vi "APU + 1 Directional Sim.vi"() -> ()   [LabVIEW 2013]
uses:
  IP Source/Version Token.ctl
  IP Source/APU/Settings.ctl
  IP Source/APU/Input.ctl
  IP Source/APU/Output.ctl
  IP Source/Directional Speed/Load Input.ctl
  IP Source/Directional Speed/Input.ctl
  IP Source/Directional Speed/Settings.ctl
  IP Source/APU/Shared Settings.ctl
  <vilib>/Platform/TimedLoop/XDataNode/timing_clust.ctl
  <vilib>/Platform/TimedLoop/XDataNode/nitl_modes.ctl
  <vilib>/Platform/TimedLoop/XDataNode/wakeup.ctl
  <vilib>/rvi/DataTransferAndStorage/Container/Common/niFpgaContainerGetUniqueNameForEmu.vi
  <vilib>/rvi/DataTransferAndStorage/Container/Common/niFpgaContainerSetEmuInfo.vi
  <vilib>/rvi/eio/common/nirviEmuReportErrorAndStop.vi
  <vilib>/rvi/Emulation/niFpgaSctlEmulationGetInTimedLoop.vi
  <vilib>/rvi/Emulation/niFpgaEmulationReportErrorSimple.vi
  <vilib>/rvi/Emulation/niFpgaGetClockAttributes.vi
  <vilib>/rvi/Emulation/niFpgaCriticalErrorInLSC.vi
  <vilib>/rvi/eio/common/nirviEmuTemplateMethod_errors.vi
  <vilib>/Platform/TimedLoop/XDataNode/XDataNode.xnode
  <vilib>/rvi/LocalResourceManager/LocalResourceManager.xnode
  <vilib>/eio/EIONode/EIONode.xnode
  <vilib>/Platform/TimedLoop/XDataNode/XDNodeRunTimeDep.lvlib
  IP Source/APU/APU.lvlib
  IP Source/Directional Speed/Directional Speed.lvlib
  IP Source/Engine Simulation Toolkit.lvlib
panel:
  in  "shared settings.my apu":T1 {"start" format="%#.15g"}
  in  "go.my apu":bool
  in  "settings.DirectionSim":T2
  in  "input.DirectionSim":T3
  in  "load input.DirectionSim":T4
  out "output.my apu":T5 caption="output"
  in  "input.my apu":T6={"desired speed"=0.0, "reset"=TRUE} caption="input"
  in  "settings.my apu":T7 caption="settings"
  in  "eps.version":T8
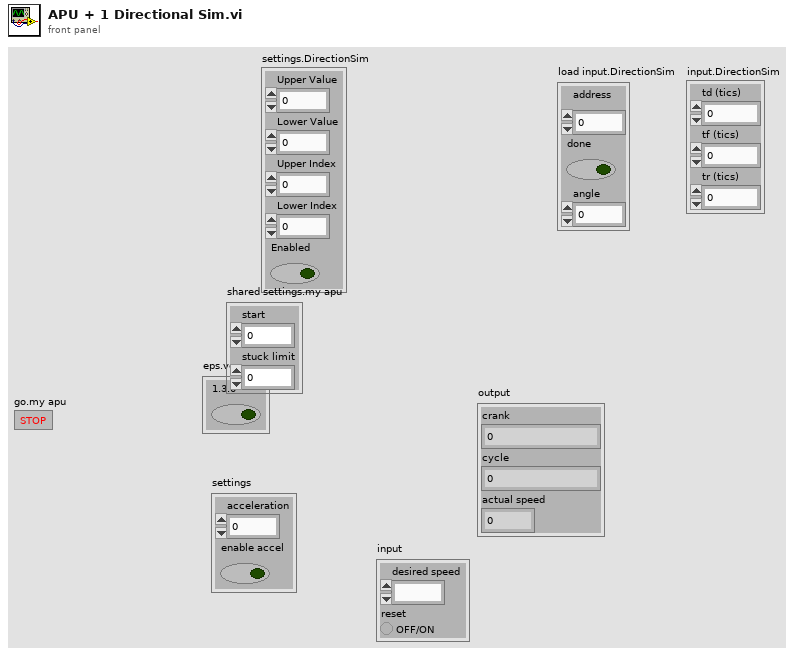
[diagram p1: front panel]
types:
  T1 = typedef "Engine Simulation Toolkit.lvlib/APU.lvlib/Shared Settings.ctl" = cluster{"start":fxp<+,17,17>, "stuck limit":fxp<+,18,18>}
  T2 = typedef "Engine Simulation Toolkit.lvlib/Directional Speed.lvlib/Settings.ctl" = cluster{"Upper Value":u16, "Lower Value":u16, "Upper Index":fxp<+,10,10>, "Lower Index":fxp<+,10,10>, "Enabled":bool}
  T3 = typedef "Engine Simulation Toolkit.lvlib/Directional Speed.lvlib/Input.ctl" = cluster{"td (tics)":u16, "tf (tics)":u16, "tr (tics)":u16}
  T4 = typedef "Engine Simulation Toolkit.lvlib/Directional Speed.lvlib/Load Input.ctl" = cluster{"address":fxp<+,10,10>, "done":bool, "angle":u16}
  T5 = typedef "Engine Simulation Toolkit.lvlib/APU.lvlib/Output.ctl" = cluster{"crank":u16, "cycle":u16, "actual speed":fxp<+/-,23,2>}
  T6 = typedef "Engine Simulation Toolkit.lvlib/APU.lvlib/Input.ctl" = cluster{"desired speed":fxp<+/-,23,2>, "reset":bool}
  T7 = typedef "Engine Simulation Toolkit.lvlib/APU.lvlib/Settings.ctl" = cluster{"acceleration":fxp<+,18,-20>, "enable accel":bool}
  T8 = typedef "Engine Simulation Toolkit.lvlib/Version Token.ctl" = cluster{"1.3.0":bool}
  T9 = typedef "XDNodeRunTimeDep.lvlib/timing_clust.ctl" = cluster{"Expected End [f-1]":u64, "Actual End [f-1]":u64, "Finished Late? [f-1]":bool, "Expected End [i-1]":u64, "Actual End [i-1]":u64, "Finished Late? [i-1]":bool, "Expected Start [i]":u64, "Actual Start [i]":u64, "Expected Start [f]":u64, "Actual Start [f]":u64, "Source Name":string, "Structure Name":string, "Period":i64, "Deadline":i64, "Offset":i64, "Start":i64, "Priority":i32, "Timeout":i32, "Mode":T10, "Wakeup Reason":T11, "Error":errorcluster, "Source Type":string, "Secondary Source Type":string, "Global End Time":u64, "Global Start Time":u64, "Frame Duration":u64, "Iteration Duration":u64, "Assigned CPU":i32, "I/O Scan Engine Mode":u32}
  T10 = typedef "XDNodeRunTimeDep.lvlib/nitl_modes.ctl" = enum32{"No Change", "Process missed periods, maintain original phase", "Discard missed periods, maintain original phase", "Process missed periods, ignore original phase", "Discard missed periods, ignore original phase"}
  T11 = typedef "XDNodeRunTimeDep.lvlib/wakeup.ctl" = enum32{"Normal", "Aborted", "Asynchronous wakeup", "Timing source error", "Timed loop error", "Timeout"}
  T12 = typedef "Engine Simulation Toolkit.lvlib/APU.lvlib/Register Bus.ctl" = cluster{"Speed":refnum<k21>, "Crank Angle":refnum<k21>, "Cycle Angle":refnum<k21>, "Crank Count":refnum<k21>, "Cycle Count":refnum<k21>, "1.25 MHz Counter":refnum<k21>, "Crank Rollover":refnum<k21>, "Cycle Rollover":refnum<k21>, "shared settings":T1}
  T13 = typedef "Engine Simulation Toolkit.lvlib/Directional Speed.lvlib/Load Data.ctl" = cluster{"max address":fxp<+,10,10>, "Memory":refnum<k21>}
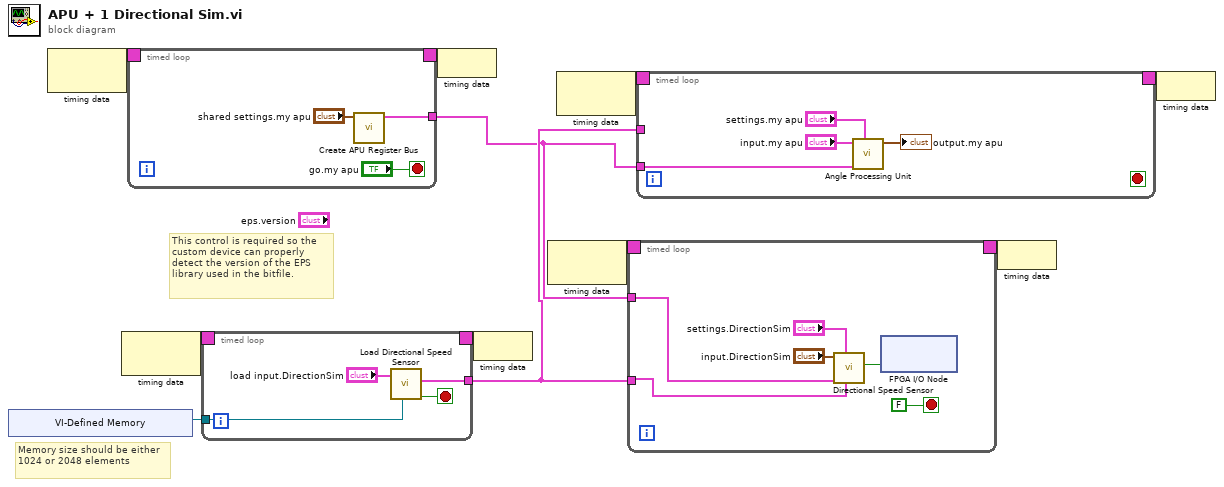
[diagram p0: block diagram]
diagram:
  # "This control is required so the custom device can properly detect the version of the EPS library used in the bitfile."
  # "Memory size should be either 1024 or 2048 elements"
  n1 = xnode "VI-Defined Memory"() -> ("Memory Out"=w9:refnum<k21>)
  n2 = node-c288() -> (w3:T9)  [unwired: 1 in]
  n3 = node-c288() -> (w11:T9)  [unwired: 1 in]
  n4 = timed-loop {
    timing: w3 -> [_]
    timing-out: [_] -> w2
    tunnel: [w14] -> w1
    stop <- "go.my apu" stop-if-true
    n5 = call "Create APU Register Bus.vi"("shared settings.<user name>"="shared settings.my apu") -> ("register bus"=w14:T12)  [unwired: 10 in]
  }
  n6 = timed-loop {
    timing: w11 -> [_]
    timing-out: [_] -> w10
    tunnel: w9 -> [w19]
    tunnel: [w18] -> w4
    stop <- w20 stop-if-true
    n7 = call "Load Directional Speed Sensor.vi"("Memory In"=w19, "load input.<user name>"="load input.DirectionSim") -> ("done"=w20:bool, "load data"=w18:T13)  [unwired: 8 in]
  }
  n8 = node-c288(w2) -> ()
  n9 = node-c288(w10) -> ()
  n10 = node-c288() -> (w8:T9)  [unwired: 1 in]
  n11 = node-c288() -> (w6:T9)  [unwired: 1 in]
  n12 = timed-loop {
    tunnel: w1 -> [w26]
    timing: w8 -> [_]
    timing-out: [_] -> w7
    tunnel: w4 -> [w25]
    stop <- FALSE stop-if-true
    n13 = call "Directional Speed Sensor.vi"("load data"=w25, "settings.<user name>"="settings.DirectionSim", "register bus"=w26, "input.<user name>"="input.DirectionSim") -> ("digial output"=w27:bool)  [unwired: 7 in]
    n14 = xnode "FPGA I/O Node"("DO0"=w27) -> ()  [unwired: 1 in, 1 out]
  }
  n15 = timed-loop {
    timing: w6 -> [_]
    timing-out: [_] -> w5
    tunnel: w1 -> [w31]
    tunnel: w4 -> [_]
    stop <- _ stop-if-true
    n16 = call "Angle Processing Unit.vi"("settings.<user name>"="settings.my apu", "register bus"=w31, "input.<user name>"="input.my apu") -> ("output.<user name>"=→"output.my apu":T5)  [unwired: 8 in]
  }
  n17 = node-c288(w7) -> ()
  n18 = node-c288(w5) -> ()
